vi "Code Coverage.vi"(10 "Selector 2":enum16{"Case 1", "Case 2", "Case 3"}(ring), 11 "Selector 1":enum16{"Case 1", "Case 2"}(ring)) -> (3 "Waveform Graph":dbl[](graph))   [LabVIEW 2023]
doc: "Demonstrates how to use the LabVIEW Unit Test Framework Toolkit to measure the percentage of diagrams that LabVIEW executes when you run a VI."
uses:
  <vilib>/Analysis/1siggen.llb/Ramp Pattern by Samples.vi
  <vilib>/Analysis/NI_AALBase.lvlib
panel:
  # "Overview: Demonstrates how to use the LabVIEW Unit Test Framework Toolkit to measure the percentage of diagrams that LabVIEW executes when you run a VI.\nRequirements: LabVIEW Full Development System, Unit Test Framework Toolkit\nInstructions:\n1.  In the Project Explorer window, click the Run Unit Tests button to run all the test files in the project.\n2.  View the test results in the Unit Test Framework Results window. Two tests pass and one test are configured to fail.\n3.  Click the Code Coverage tab in the Unit Test Framework Results window to display code coverage details.\n4.  In the Project Explorer window, double-click the test files to display the Test Properties dialog boxes, in which you can find details for each test file.\n5.\tRead the comments on the block diagram of this VI to understand how the LabVIEW Unit Test Framework Toolkit calculates code coverage."
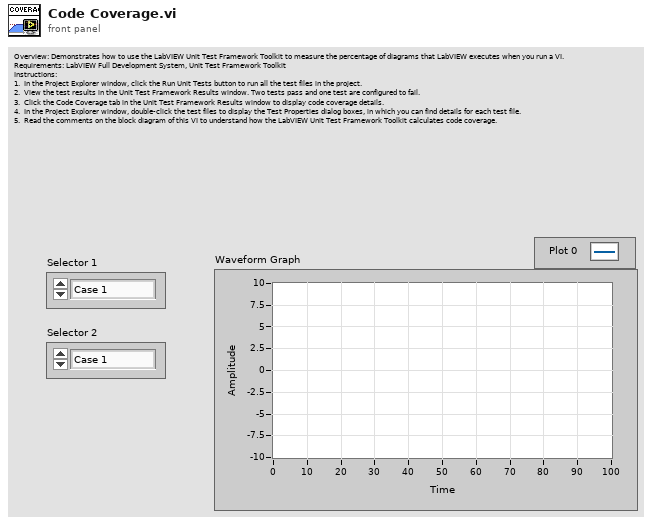
[diagram p1: front panel]
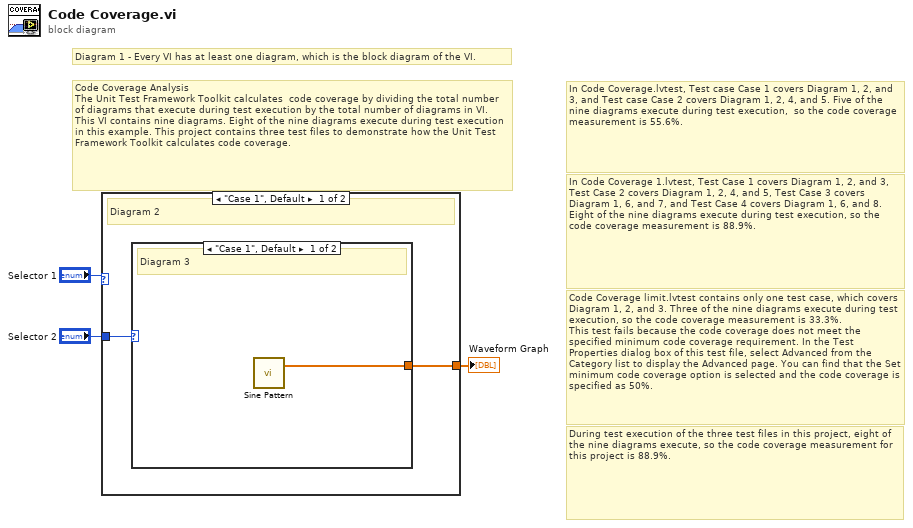
[diagram p0: block diagram]
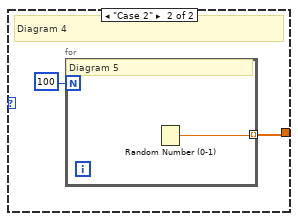
[diagram p2: hidden frame]
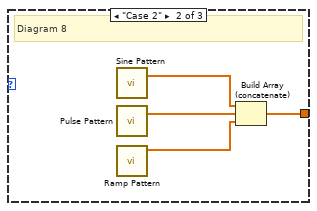
[diagram p4: hidden frame]
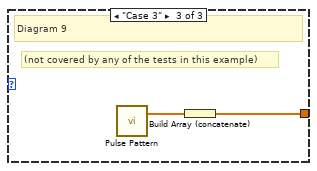
[diagram p5: hidden frame]
diagram:
  # "During test execution of the three test files in this project, eight of the nine diagrams execute, so the code coverage measurement for this project is 88.9%."
  # "Code Coverage limit.lvtest contains only one test case, which covers Diagram 1, 2, and 3. Three of the nine diagrams execute during test execution, so the code coverage measurement is 33.3%.\nThis test fails because the code coverage does not meet the specified minimum code coverage requirement. In the Test Properties dialog box of this test file, select Advanced from the Category list to display the Advanced page. You can find that the Set minimum code coverage option is selected and the code coverage is specified as 50%."
  # "In Code Coverage 1.lvtest, Test Case 1 covers Diagram 1, 2, and 3, Test Case 2 covers Diagram 1, 2, 4, and 5, Test Case 3 covers Diagram 1, 6, and 7, and Test Case 4 covers Diagram 1, 6, and 8. Eight of the nine diagrams execute during test execution, so the code coverage measurement is 88.9%."
  # "In Code Coverage.lvtest, Test case Case 1 covers Diagram 1, 2, and 3, and Test case Case 2 covers Diagram 1, 2, 4, and 5. Five of the nine diagrams execute during test execution,  so the code coverage measurement is 55.6%."
  # "Code Coverage Analysis\nThe Unit Test Framework Toolkit calculates  code coverage by dividing the total number of diagrams that execute during test execution by the total number of diagrams in VI. This VI contains nine diagrams. Eight of the nine diagrams execute during test execution in this example. This project contains three test files to demonstrate how the Unit Test Framework Toolkit calculates code coverage."
  # "Diagram 1 - Every VI has at least one diagram, which is the block diagram of the VI."
  n1 = case shown="\"Case 1\", Default" "Selector 1" {
    tunnel: "Selector 2" -> [w5 w11]
    tunnel: [w4 w10] -> w1
    frame "Case 1", Default {
      # "Diagram 2"
      n2 = case shown="\"Case 1\", Default" w5 {
        tunnel: [w6 w7] -> w4
        frame "Case 1", Default {
          # "Diagram 3"
          n3 = call <vilib>:"Sine Pattern.vi"() -> ("Sinusoidal Pattern"=w6:dbl[])  [unwired: 4 in, 1 out]
        }
        frame "Case 2" {
          # "Diagram 4"
          n4 = for {
            N: 100 -> [_]
            tunnel: [w9] -> w7 mode=indexing
            # "Diagram 5"
            n5 = Random Number (0-1)() -> (number: 0 to 1=w9:dbl)
          }
        }
      }
    }
    frame "Case 2" {
      # "Diagram 6"
      n6 = case shown="\"Case 1\", Default" w11 {
        tunnel: [_ w12 w16] -> w10
        frame "Case 1", Default {
          # "Diagram 7"
        }
        frame "Case 2" {
          # "Diagram 8"
          n7 = call <vilib>:"Sine Pattern.vi"() -> ("Sinusoidal Pattern"=w15:dbl[])  [unwired: 4 in, 1 out]
          n8 = call <vilib>:"Pulse Pattern.vi"() -> ("Pulse Pattern"=w14:dbl[])  [unwired: 4 in, 1 out]
          n9 = call-poly <vilib>:"Ramp Pattern.vi"() -> ("Ramp Pattern"=w13:dbl[])  [unwired: 10 in, 1 out]
          n10 = Build Array (concatenate)(w15, w14, w13) -> (w12:dbl[])
        }
        frame "Case 3" {
          # "(not covered by any of the tests in this example)"
          # "Diagram 9"
          n11 = call <vilib>:"Pulse Pattern.vi"() -> ("Pulse Pattern"=w17:dbl[])  [unwired: 4 in, 1 out]
          n12 = Build Array (concatenate)(w17) -> (w16:dbl[])
        }
      }
    }
  }
  "Waveform Graph" <- w1
